vi "Send Polling Interval.vi"(7 "Message Priority (Normal)":T1=enum."Normal", 8 "error in (no error)":errorcluster, 10 "Polling Interval":dbl[unit], 11 "Message Enqueuer":refnum<class "Message Enqueuer.lvclass">) -> (0 "error out":errorcluster, 3 "Message Enqueuer out":refnum<class "Message Enqueuer.lvclass">)   [LabVIEW 2015, in "CS++BaseActor.lvlib" / "Polling Interval Msg.lvclass"]
doc: "Sends the <B>CS++BaseActor.lvlib:Polling Interval Msg.lvclass</B> message.\n\n<B>CS++BaseActor.lvlib:CS++BaseActor.lvclass:Polling Interval.vi</B> Description:\n\nIntervall for periodic actions.\n\n<b>Attention:</b> Be aware of message pileup if intervall is too short."
uses:
  Polling Interval Msg.lvclass
  <vilib>/ActorFramework/Message Enqueuer/Message Enqueuer.lvclass
  <vilib>/ActorFramework/Message Enqueuer/Message Priority.ctl
  Polling Interval Msg.lvclass/Polling Interval Msg.ctl
  <vilib>/ActorFramework/Message Enqueuer/Message Enqueuer.lvclass/Message Enqueuer.ctl
  <vilib>/ActorFramework/Message Priority Queue/Priority Enqueue.vi
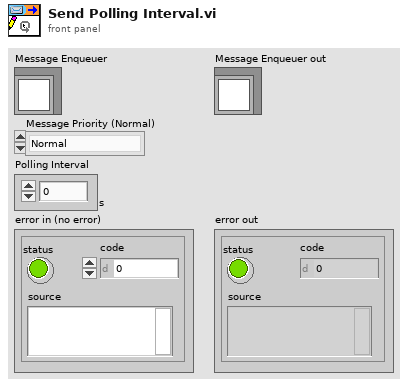
[diagram p1: front panel]
types:
  T1 = typedef "Actor Framework.lvlib/Message Enqueuer.lvclass/Message Priority.ctl" = enum16{"Low", "Normal", "High"}
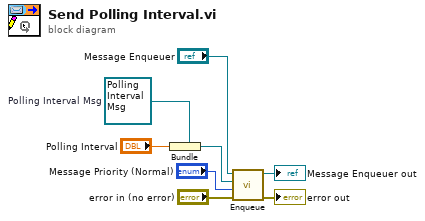
[diagram p0: block diagram]
diagram:
  w2 = refnum<class "Polling Interval Msg.lvclass"> refnum  # Polling Interval Msg
  n1 = Bundle(cluster=w2, "Polling Interval") -> (w5:refnum<class "Polling Interval Msg.lvclass">)
  n2 = call <vilib>:"Enqueue.vi"("error in (no error)"="error in (no error)", "Message Priority (Normal)"="Message Priority (Normal)", "Message"=w5, "Message Enqueuer in"="Message Enqueuer") -> ("error out"=→"error out":errorcluster, "Message Enqueuer out"=→"Message Enqueuer out":refnum<class "Message Enqueuer.lvclass">)  [unwired: 6 in]
